vi "Calculate_Desired_Flowrates.vi"(8 "Strength (% by volume)":dbl=3.0 format="%.2f", 9 "Carrier_2 Q (l/min)":dbl=20.0 format="%.2f", 10 "Carrier_1 Q (l/min)":dbl=20.0 format="%.2f") -> (0 "Error Message":string, 1 "Trace Q l/min":dbl format="%.2f", 2 "Carrier 2 l/min":dbl format="%.2f", 3 "Carrier 1 l/min":dbl format="%.2f", 4 "Carrier Info":string)   [LabVIEW 2021]
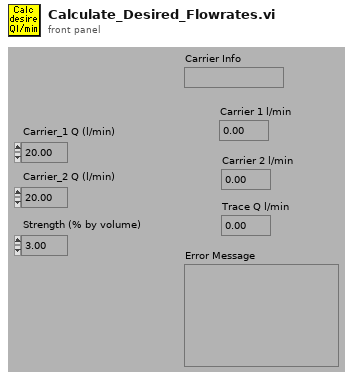
[diagram p1: front panel]
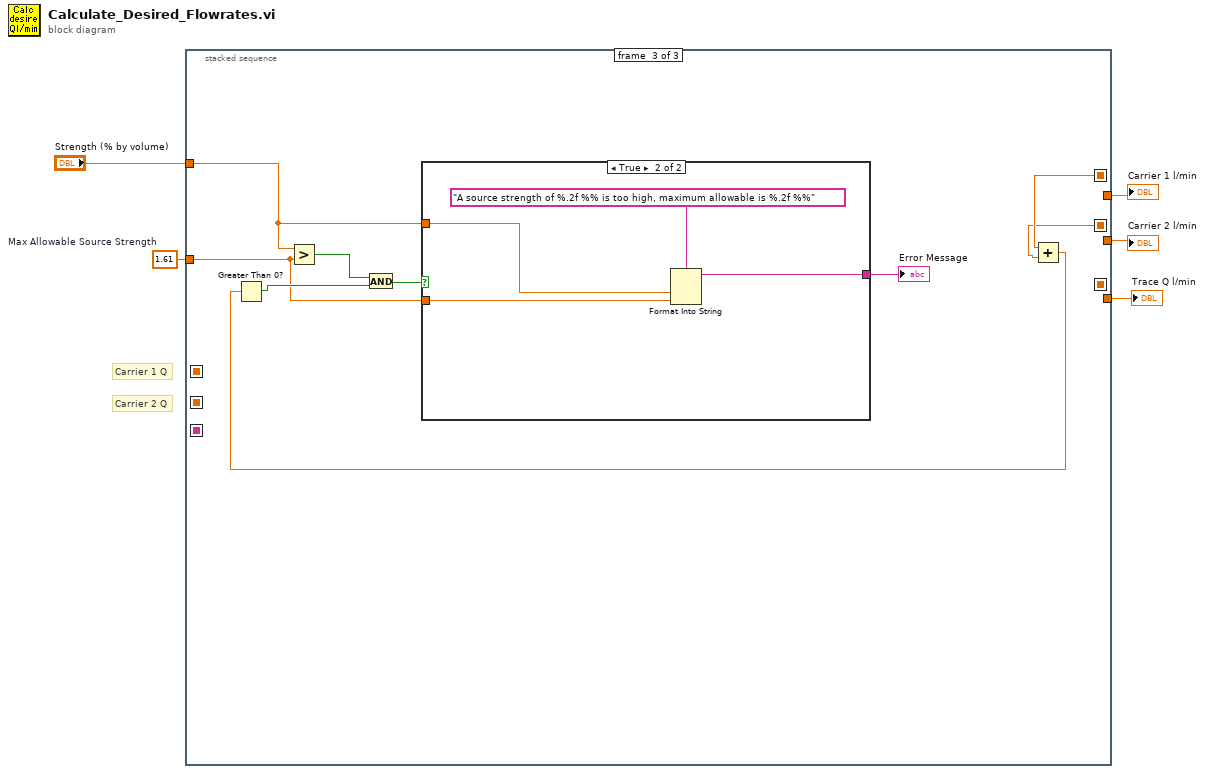
[diagram p0: block diagram]
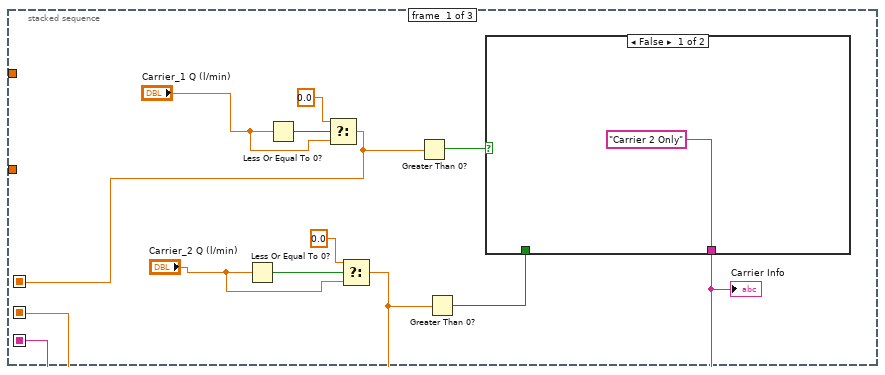
[diagram p2: hidden frame]
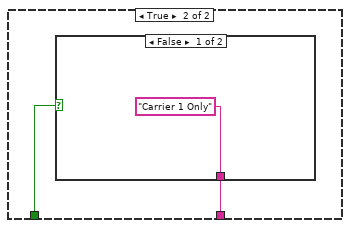
[diagram p3: hidden frame]
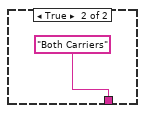
[diagram p4: hidden frame]
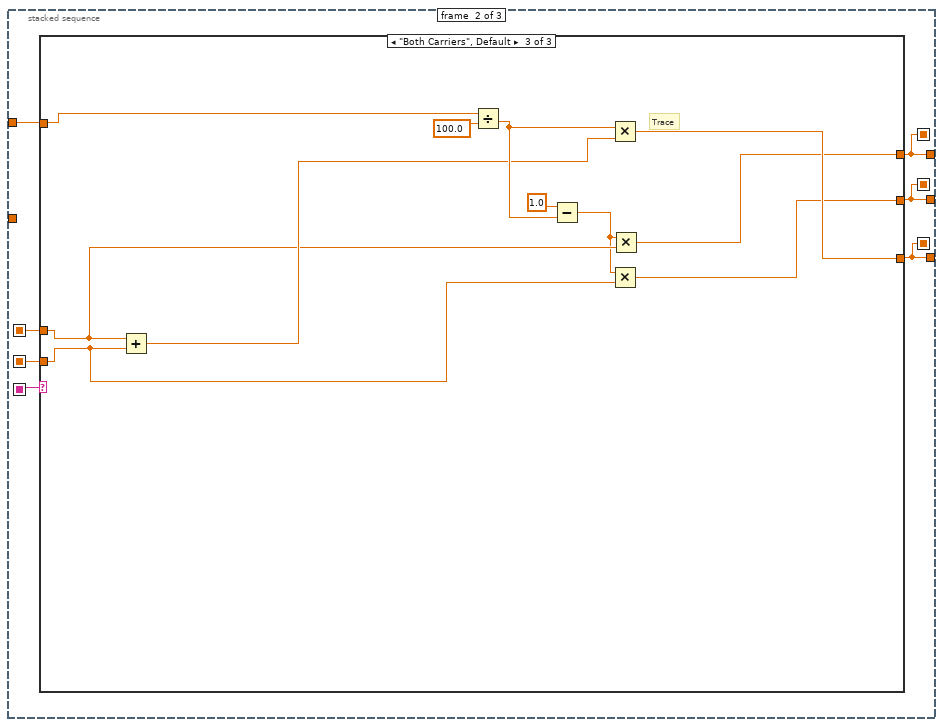
[diagram p5: hidden frame]
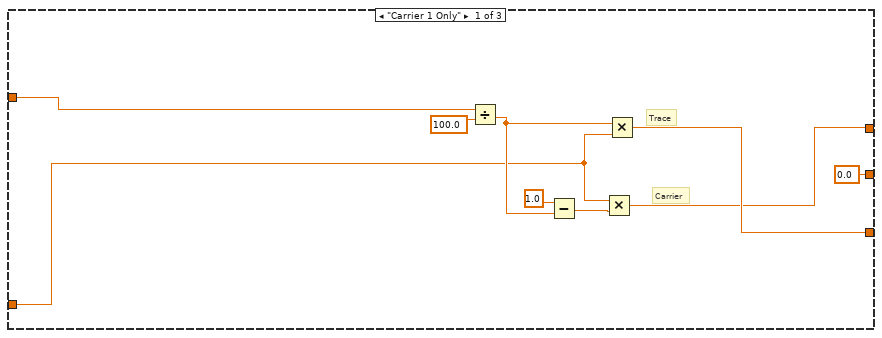
[diagram p6: hidden frame]
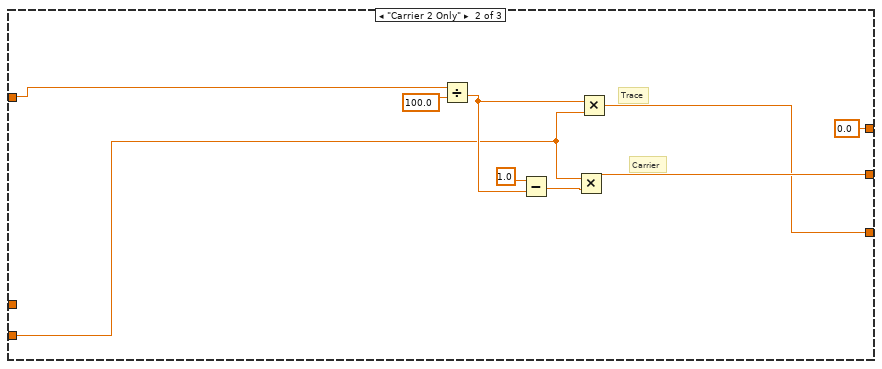
[diagram p7: hidden frame]
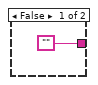
[diagram p8: hidden frame]
diagram:
  w1 = 1.61  # Max Allowable Source Strength
  # "Carrier 2 Q"
  # "Carrier 1 Q"
  n1 = stacked-sequence {
    seq-local: [_ w25 _] -> [_ _ w62]
    seq-local: [_ w26 _] -> [_ _ w61]
    seq-local: [_ w27 _] -> [_ _ _]
    seq-local: [w10 _ _] -> [_ w23 _]
    seq-local: [w9 _ _] -> [_ w22 _]
    seq-local: [w6 _ _] -> [_ w24 _]
    tunnel: "Strength (% by volume)" -> [_ w28 w63]
    tunnel: [_ w27 _] -> w4
    tunnel: [_ w25 _] -> w3
    tunnel: [_ w26 _] -> w2
    tunnel: w1 -> [_ _ w58]
    frame #0 {
      n2 = Less Or Equal To 0?(x="Carrier_2 Q (l/min)") -> (x <= 0?=w12:bool)
      n3 = Less Or Equal To 0?(x="Carrier_1 Q (l/min)") -> (x <= 0?=w16:bool)
      n4 = Select(t=0.0, s=w16, f="Carrier_1 Q (l/min)") -> (s? t:f=w10:dbl)
      n5 = Select(t=0.0, s=w12, f="Carrier_2 Q (l/min)") -> (s? t:f=w9:dbl)
      n6 = Greater Than 0?(x=w10) -> (x > 0?=w8:bool)
      n7 = Greater Than 0?(x=w9) -> (x > 0?=w7:bool)
      n8 = case shown="False" w8 {
        tunnel: w7 -> [_ w19]
        tunnel: ["Carrier 2 Only" w18] -> w6
        frame False {
        }
        frame True {
          n9 = case shown="False" w19 {
            tunnel: ["Carrier 1 Only" "Both Carriers"] -> w18
            frame False {
            }
            frame True {
            }
          }
        }
      }
      "Carrier Info" <- w6
    }
    frame #1 {
      n10 = case shown="\"Both Carriers\", Default" w24 {
        tunnel: w28 -> [w34 w42 w54]
        tunnel: [0.0 ("Qc2") w41 w47] -> w26
        tunnel: [w32 w40 w53] -> w27
        tunnel: [w31 0.0 ("Qc1") w48] -> w25
        tunnel: w23 -> [w29 _ w51]
        tunnel: w22 -> [_ w38 w49]
        frame "Carrier 1 Only" {
          # "Carrier"
          # "Trace"
          n11 = Divide(x=w34, y=100.0) -> (x/y=w33:dbl)
          n12 = Subtract(x=1.0, y=w33) -> (x-y=w37:dbl)
          n13 = Multiply(x=w29, y=w37) -> (x*y=w31:dbl)
          n14 = Multiply(x=w33, y=w29) -> (x*y=w32:dbl)
        }
        frame "Carrier 2 Only" {
          # "Carrier"
          # "Trace"
          n15 = Divide(x=w42, y=100.0) -> (x/y=w43:dbl)
          n16 = Subtract(x=1.0, y=w43) -> (x-y=w46:dbl)
          n17 = Multiply(x=w38, y=w46) -> (x*y=w41:dbl)
          n18 = Multiply(x=w43, y=w38) -> (x*y=w40:dbl)
        }
        frame "Both Carriers", Default {
          # "Trace"
          n19 = Add(x=w51, y=w49) -> (x+y=w52:dbl)
          n20 = Divide(x=w54, y=100.0) -> (x/y=w55:dbl)
          n21 = Subtract(x=1.0, y=w55) -> (x-y=w50:dbl)
          n22 = Multiply(x=w55, y=w52) -> (x*y=w53:dbl)
          n23 = Multiply(x=w50, y=w49) -> (x*y=w47:dbl)
          n24 = Multiply(x=w50, y=w51) -> (x*y=w48:dbl)
        }
      }
    }
    frame #2 {
      n25 = Greater?(x=w63, y=w58) -> (0:w66:bool)
      n26 = Add(x=w62, y=w61) -> (x+y=w60:dbl)
      n27 = Greater Than 0?(x=w60) -> (x > 0?=w65:bool)
      n28 = And(x=w66, y=w65) -> (x .and. y?=w64:bool)
      n29 = case shown="True" w64 {
        tunnel: w63 -> [_ w71]
        tunnel: w58 -> [_ w69]
        tunnel: ["" w68] -> w59
        frame False {
        }
        frame True {
          n30 = Format Into String(format string="A source strength of %.2f %% is too high, maximum allowable is %.2f %%" ("Format String"), w71, w69) -> (resulting string=w68:string)  [unwired: 2 in, 1 out]
        }
      }
      "Error Message" <- w59
    }
  }
  "Carrier 1 l/min" <- w3
  "Carrier 2 l/min" <- w2
  "Trace Q l/min" <- w4
